vi "Enqueue Error.vi"(8 "Error In":errorcluster, 9 "Index":u32, 11 "HWSync Message Queue":refnum<queue>) -> (0 "dup Error Out":errorcluster)   [LabVIEW 2014, in "HWSyncLoop.lvlib"]
uses:
  HWSyncLoop.lvlib
  APIs/Message Queue/Message Cluster.ctl
  APIs/Message Queue/Enqueue Message (Single).vi
  APIs/Message Queue/WINFAS 2 Message Queue.lvlib
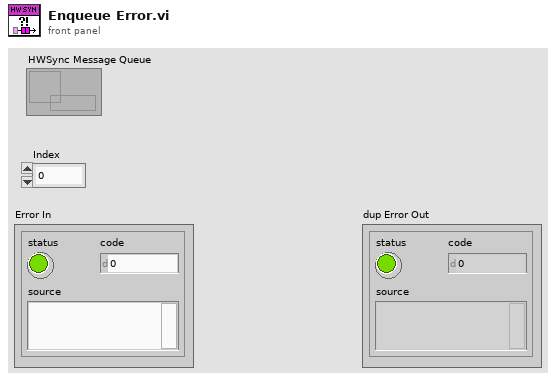
[diagram p1: front panel]
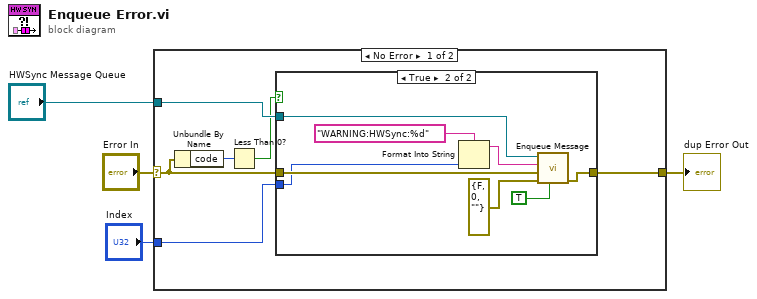
[diagram p0: block diagram]
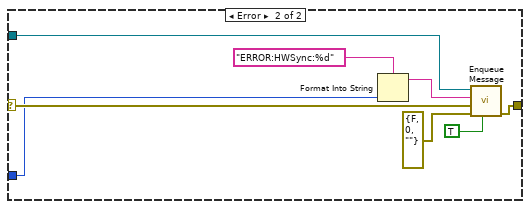
[diagram p3: hidden frame]
diagram:
  n1 = case shown="No Error" "Error In" {
    selector: "Error In" -> [w9 w26]
    tunnel: [w7 w24] -> w2
    tunnel: "HWSync Message Queue" -> [w8 w27]
    tunnel: "Index" -> [w5 w20]
    frame No Error {
      n2 = Unbundle By Name(w9) -> ("code"=w10:i32)
      n3 = Less Than 0?(x=w10) -> (x < 0?=w6:bool)
      n4 = case shown="True" w6 {
        tunnel: w9 -> [w11 w15]
        tunnel: w8 -> [_ w14]
        tunnel: [w11 w13] -> w7
        tunnel: w5 -> [_ w12]
        frame False {
        }
        frame True {
          n5 = Format Into String(format string="WARNING:HWSync:%d" ("Message"), w12) -> (resulting string=w16:string)  [unwired: 2 in, 1 out]
          n6 = call-poly "Enqueue Message.vi"("Priority Message? (F)"=TRUE, "error in (no error)"=errorcluster {"status"=FALSE, "code"=0, "source"=""} ("error constant"), "Message Data"=w15, "Message"=w16, "Message Queue"=w14) -> ("error out"=w13:errorcluster)  [unwired: 5 in, 1 out]
        }
      }
    }
    frame Error {
      n7 = Format Into String(format string="ERROR:HWSync:%d" ("Message"), w20) -> (resulting string=w21:string)  [unwired: 2 in, 1 out]
      n8 = call-poly "Enqueue Message.vi"("Priority Message? (F)"=TRUE, "error in (no error)"=errorcluster {"status"=FALSE, "code"=0, "source"=""} ("error constant"), "Message Data"=w26, "Message"=w21, "Message Queue"=w27) -> ("error out"=w24:errorcluster)  [unwired: 5 in, 1 out]
    }
  }
  "dup Error Out" <- w2
